vi "Turret_Globals.vi"() -> ()   [LabVIEW 2019]
uses:
  Turret_Cluster.ctl
panel:
  in  "Turret_Flywheel_Left":string="Turret_Flywheel_Left"
  in  "Turret_Execute_Notifier":refnum<notifier>
  in  "Turret_Set_Notifier":refnum<notifier>
  in  "Turret_Execute_Ref":string="Turret_Execute_Ref"
  in  "Turret_Set_Ref":string="Turret_Set_Ref"
  in  "Turret_Flywheel_Right":string="Turret_Flywheel_Right"
  in  "Turret_Spin":string="Turret_Spin"
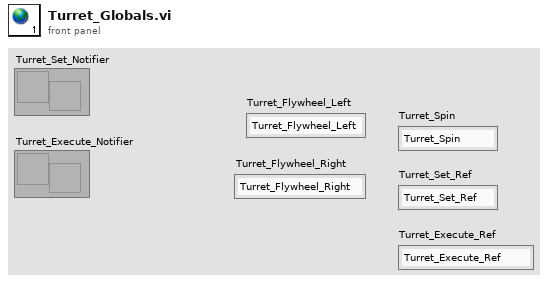
[diagram p1: front panel]
diagram:
